vi "MiniReader.vi"() -> ()   [LabVIEW 2017]
uses:
  <vilib>/S3DK/PMU Recorder Light/PMU Recorder Light.lvlib
panel:
  out "error out":errorcluster
  in  "error in (no error)":errorcluster
  out "Buffer Active":bool
  out "Configuration File Received":bool
  out "Connected":bool
  out "Status Loop":bool
  out "Error":bool
  in  "Tab Control":T1(tab)
  out "Frequency":waveform(sgl)[](graph)
  out "Phasor_Mag":waveform(sgl)[](graph) caption="Frequency"
  out "Phasor_Ang":waveform(sgl)[](graph) caption="Frequency"
  out "Timestamp":timestamp[](array[timestamp])
  out "Analog Signals":sgl[][](array[numeric])
  out "Phasor Signals":csg[][](array[numeric])
  out "Digital Signals":bool[][](array[boolean])
  out "Has New Data?":bool
  out "Timed Loop":bool
  out "Signal Names":T2
  in  "Refresh Rate":i64(ring)=200 items=["50 Hz"=20, "20 Hz"=50, "10 Hz"=100, "5 Hz"=200, "2 Hz"=500, "1 Hz"=1000, "Every 2 sec"=2000, "Every 5 sec"=5000, "Every 10 sec"=10000, "Every minute"=60000]
  out "Quitting":bool
  in  "Activate PRL Read":bool=TRUE
  out "Execution Loop":bool
  out "Status":string
  in  "Channel Selector":bool
  in  "PRL Visible":bool
  in  "Quit":bool
  out "Event Loop":bool
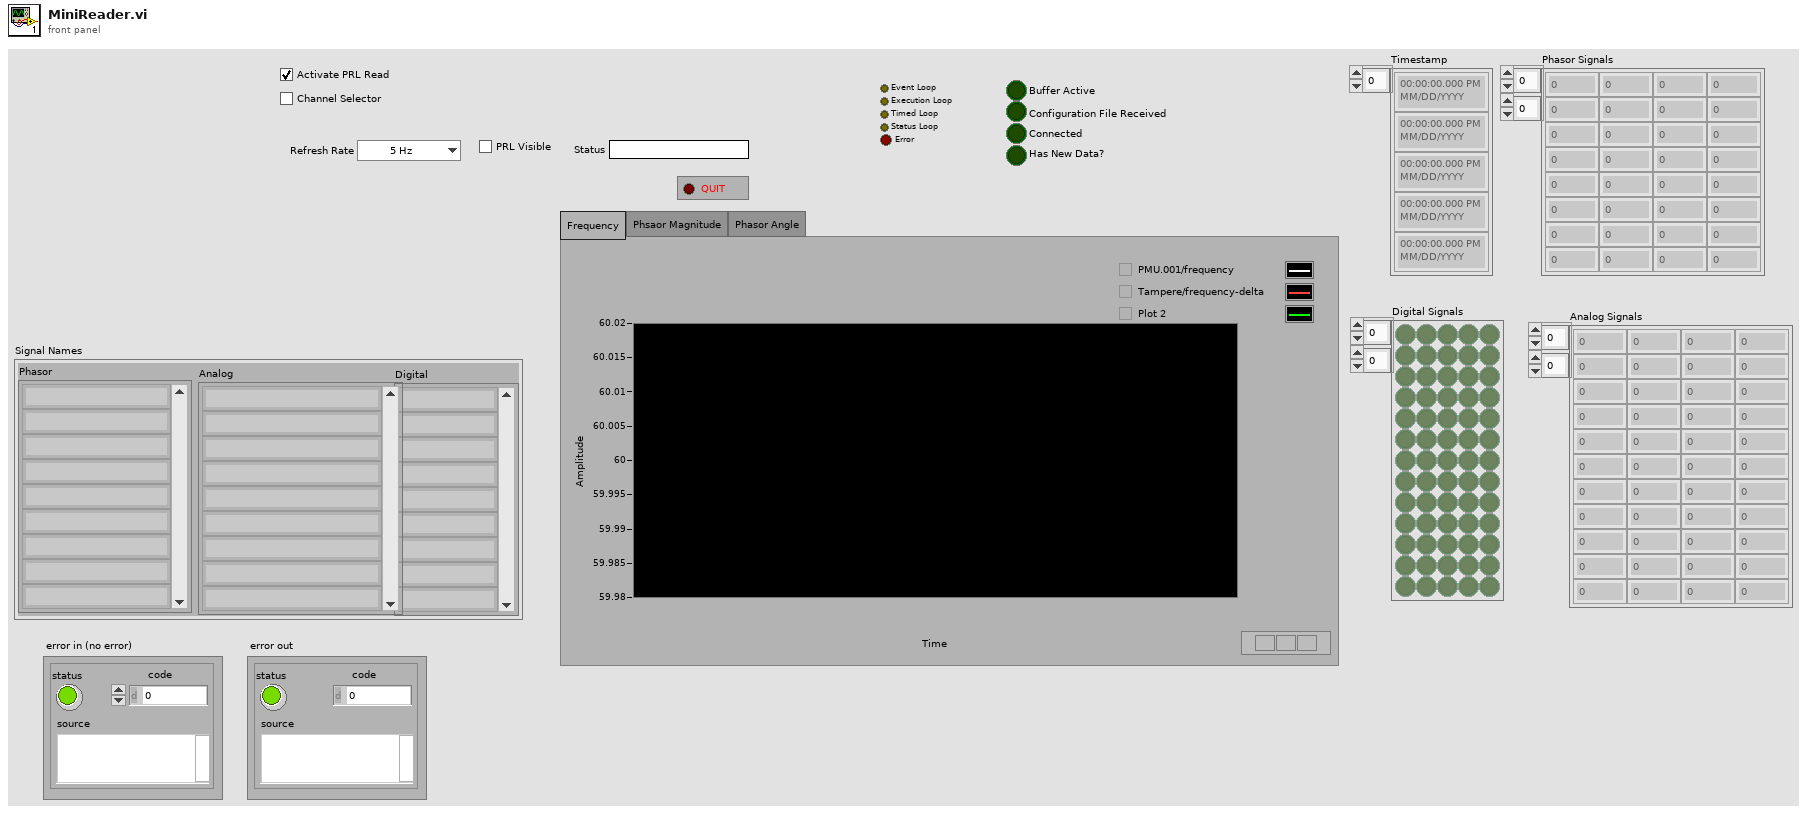
[diagram p1: front panel]
types:
  T1 = enum32{"Frequency", "Phsaor Magnitude", "Phasor Angle"}
  T2 = cluster{"Phasor":string[], "Analog":string[], "Digital":string[]}
  T3 = enum16{"Run", "Startup", "Get Status", "Pause", "Continue", "Shutdown", "Abort", "Open Panel", "Close Panel"}
  T4 = enum32{"Invalid", "Standard", "Closed", "Hidden", "Minimized", "Maximized"}
  T5 = enum16{"Filter Signals", "Get All Signal Names", "Select Signals on Name", "Select Frequency Only", "Get Selected Signal Names"}
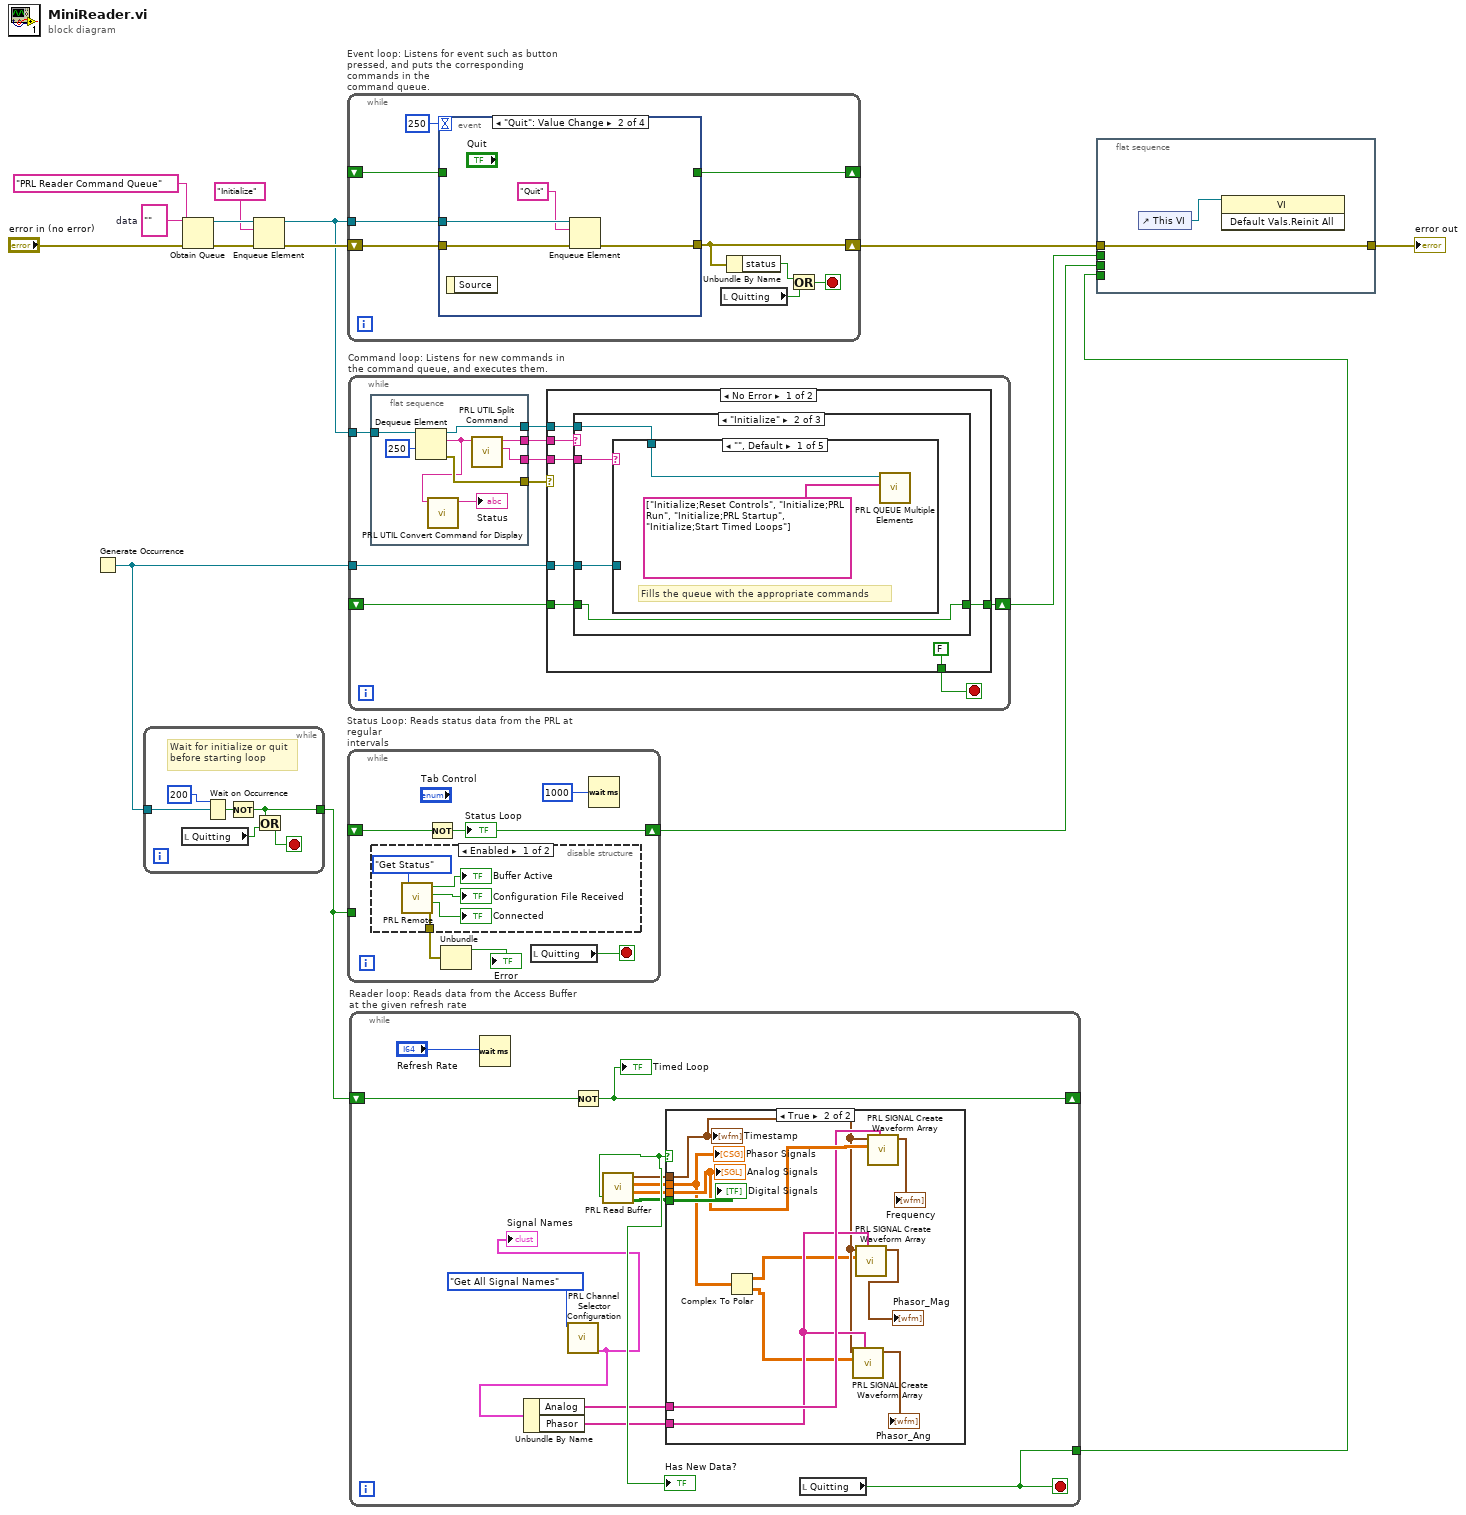
[diagram p0: block diagram]
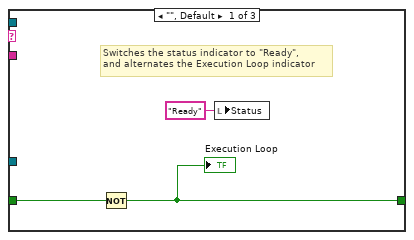
[diagram p4: hidden frame]
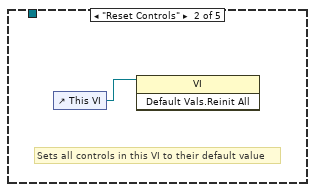
[diagram p5: hidden frame]
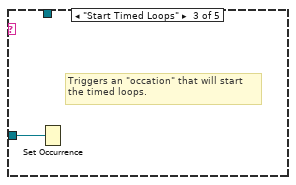
[diagram p6: hidden frame]
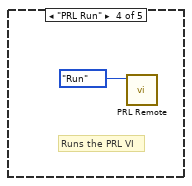
[diagram p7: hidden frame]
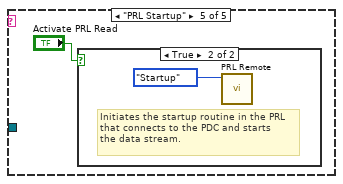
[diagram p8: hidden frame]
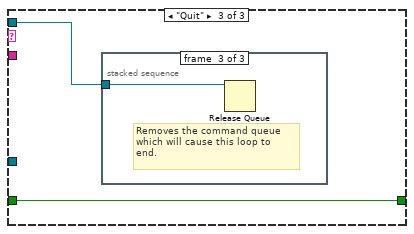
[diagram p10: hidden frame]
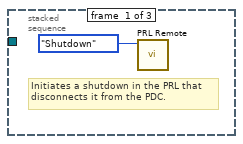
[diagram p11: hidden frame]
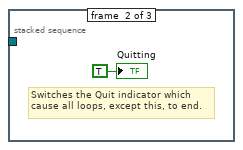
[diagram p12: hidden frame]
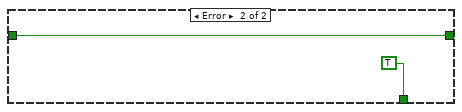
[diagram p13: hidden frame]
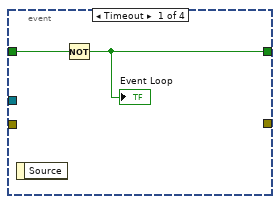
[diagram p14: hidden frame]
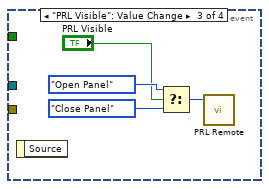
[diagram p15: hidden frame]
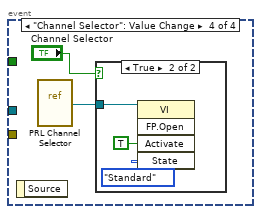
[diagram p16: hidden frame]
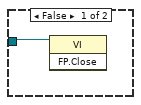
[diagram p17: hidden frame]
diagram:
  w15 = ""  # data
  n1 = Generate Occurrence() -> (w10:refnum<k4>)
  n2 = while {
    tunnel: w10 -> [w21]
    tunnel: [w16] -> w8
    stop <- w17 stop-if-true
    # "Wait for initialize or quit\nbefore starting loop"
    n3 = local read "Quitting"() -> (w18:bool)
    n4 = Wait on Occurrence(2:w21, 3:200 ("ms timeout (-1)")) -> (0:w19:bool)  [unwired: 1 in]
    n5 = Not(x=w19) -> (.not. x?=w16:bool)
    n6 = Or(x=w16, y=w18) -> (x .or. y?=w17:bool)
  }
  n7 = Obtain Queue(name (unnamed)="PRL Reader Command Queue", element data type=w15, error in (no error)="error in (no error)") -> (queue out=w14:refnum<queue>, error out=w13:errorcluster)  [unwired: 2 in, 1 out]
  n8 = Enqueue Element(queue=w14, element="Initialize", error in (no error)=w13) -> (queue out=w9:refnum<queue>, error out=w12:errorcluster)  [unwired: 1 in, 1 out]
  n9 = while "Event loop: Listens for event such as button pressed, and puts the corresponding commands in the\ncommand queue." {
    shift-right: [w27] -> w6
    shift-left: w12 -> [w29]
    tunnel: w9 -> [w30]
    shift-right: [w22] -> _
    shift-left: _ -> [w23]
    stop <- w28 stop-if-true
    n10 = event shown="[1] \"Quit\": Value Change" {
      selector: _ -> [_ _ _ _]
      dyn-events: _ -> [_ _ _ _]
      timeout: 250 -> [_ _ _ _]
      tunnel: w30 -> [_ w35 _ _]
      tunnel: w29 -> [_ w36 _ _]
      tunnel: [_ w34 _ _] -> w27
      tunnel: w23 -> [w32 _ _ _]
      tunnel: [w31 _ _ _] -> w22
      event Timeout {
        n11 = event-data() -> ()  [unwired: 1 in, 1 out]
        n12 = Not(x=w32) -> (.not. x?=w31:bool)
        "Event Loop" <- w31
      }
      event "Quit": Value Change {
        n13 = event-data() -> ()  [unwired: 1 in, 1 out]
        n14 = Enqueue Element(queue=w35, element="Quit", error in (no error)=w36) -> (error out=w34:errorcluster)  [unwired: 1 in, 2 out]
      }
      event "PRL Visible": Value Change {
        n15 = event-data() -> ()  [unwired: 1 in, 1 out]
        n16 = Select(t=T3."Open Panel" ("Action"), s="PRL Visible", f=T3."Close Panel" ("Action")) -> (s? t:f=w37:T3)
        n17 = call <vilib>:"PRL Remote.vi"("Action"=w37) -> ()  [unwired: 5 in, 6 out]
      }
      event "Channel Selector": Value Change {
        n18 = event-data() -> ()  [unwired: 1 in, 1 out]
        n19 = vi-ref <vilib>:"PRL Channel Selector.vi"() -> (w42:refnum<vi>)
        n20 = case shown="True" "Channel Selector" {
          tunnel: w42 -> [w43 w46]
          frame False {
            n21 = invoke class="VI" method="FP.Close"(reference=w43) -> ()  [unwired: 2 in, 3 out]
          }
          frame True {
            n22 = invoke class="VI" method="FP.Open"(reference=w46, "Activate"=TRUE ("Activate?"), "State"=T4."Standard") -> ()  [unwired: 2 in, 5 out]
          }
        }
      }
    }
    n23 = local read "Quitting"() -> (w24:bool)
    n24 = Unbundle By Name(w27) -> ("status"=w26:bool)
    n25 = Or(x=w26, y=w24) -> (x .or. y?=w28:bool)
  }
  n26 = while "Status Loop: Reads status data from the PRL at regular\nintervals" {
    tunnel: w8 -> [_]
    shift-right: [w50] -> w4
    shift-left: _ -> [w51]
    stop <- w52 stop-if-true
    n27 = disable-structure shown="Enabled" {
      disable-tunnel: [w53 _] -> w49
      frame Enabled {
        n28 = call <vilib>:"PRL Remote.vi"("Action"=T3."Get Status") -> ("error out"=w53:errorcluster, "Connected"=→"Connected":bool, "Configuration File Received"=→"Configuration File Received":bool, "Buffer Active"=→"Buffer Active":bool)  [unwired: 5 in, 2 out]
      }
      frame Disabled {
      }
    }
    n29 = Not(x=w51) -> (.not. x?=w50:bool)
    "Status Loop" <- w50
    n30 = Unbundle(w49) -> ("status"=→"Error":bool)  [unwired: 2 out]
    n31 = local read "Quitting"() -> (w52:bool)
    n32 = Wait (ms)(milliseconds to wait=i64 1000 ("Period")) -> ()  [unwired: 1 out]
  }
  n33 = while "Command loop: Listens for new commands in the command queue, and executes them." {
    tunnel: w9 -> [w66]
    tunnel: w10 -> [w63]
    shift-right: [w58] -> w5
    shift-left: _ -> [w59]
    stop <- w61 stop-if-true
    n34 = flat-sequence {
      tunnel: w66 -> [w74]
      tunnel: [w73] -> w65
      tunnel: [w72] -> w64
      tunnel: [w70] -> w62
      tunnel: [w67] -> w60
      frame #0 {
        n35 = Dequeue Element(queue=w74, timeout in ms (-1)=250) -> (queue out=w72:refnum<queue>, element=w69:string, error out=w73:errorcluster)  [unwired: 1 in, 1 out]
        n36 = call <vilib>:"PRL UTIL Convert Command for Display.vi"("Command In"=w69) -> ("Command Out"=→"Status":string)  [unwired: 10 in]
        n37 = call <vilib>:"PRL UTIL Split Command.vi"("Command"=w69) -> ("Parameters"=w67:string, "Command Out"=w70:string)  [unwired: 9 in]
      }
    }
    n38 = case shown="No Error" w65 {
      tunnel: w62 -> [w81 _]
      tunnel: w64 -> [w80 _]
      tunnel: w63 -> [w79 _]
      tunnel: [FALSE TRUE] -> w61
      tunnel: w60 -> [w77 _]
      tunnel: w59 -> [w76 w101]
      tunnel: [w75 w101] -> w58
      frame No Error {
        n39 = case shown="\"Initialize\"" w81 {
          tunnel: w80 -> [_ w87 w96]
          tunnel: w79 -> [_ w86 _]
          tunnel: w77 -> [_ w88 _]
          tunnel: w76 -> [w83 w85 w97]
          tunnel: [w82 w85 w97] -> w75
          frame "", Default {
            # "Switches the status indicator to \"Ready\",\nand alternates the Execution Loop indicator"
            n40 = Not(x=w83) -> (.not. x?=w82:bool)
            "Execution Loop" <- w82
            n41 = local write "Status"("Ready" ("Status")) -> ()
          }
          frame "Initialize" {
            n42 = case shown="\"\", Default" w88 {
              tunnel: w87 -> [w90 _ _ _ _]
              tunnel: w86 -> [_ _ w92 _ _]
              frame "", Default {
                # "Fills the queue with the appropriate commands"
                n43 = call <vilib>:"PRL QUEUE Multiple Elements.vi"("Elements to Add"=string[] ["Initialize;Reset Controls", "Initialize;PRL Run", "Initialize;PRL Startup", "Initialize;Start Timed Loops"], "queue"=w90) -> ()  [unwired: 8 in, 2 out]
              }
              frame "Reset Controls" {
                # "Sets all controls in this VI to their default value"
                n44 = control-ref of="This VI"() -> (w91:refnum<vi>)
                n45 = invoke class="VI" method="Default Vals.Reinit All"(reference=w91) -> ()  [unwired: 2 in, 3 out]
              }
              frame "Start Timed Loops" {
                # "Triggers an \"occation\" that will start \nthe timed loops."
                n46 = Set Occurrence(w92) -> ()
              }
              frame "PRL Run" {
                # "Runs the PRL VI"
                n47 = call <vilib>:"PRL Remote.vi"("Action"=T3."Run") -> ()  [unwired: 5 in, 6 out]
              }
              frame "PRL Startup" {
                n48 = case shown="True" "Activate PRL Read" {
                  frame False {
                  }
                  frame True {
                    # "Initiates the startup routine in the PRL\nthat connects to the PDC and starts\nthe data stream."
                    n49 = call <vilib>:"PRL Remote.vi"("Action"=T3."Startup") -> ()  [unwired: 5 in, 6 out]
                  }
                }
              }
            }
          }
          frame "Quit" {
            n50 = stacked-sequence {
              tunnel: w96 -> [_ _ w100]
              frame #0 {
                # "Initiates a shutdown in the PRL that\ndisconnects it from the PDC."
                n51 = call <vilib>:"PRL Remote.vi"("Action"=T3."Shutdown") -> ()  [unwired: 5 in, 6 out]
              }
              frame #1 {
                # "Switches the Quit indicator which\ncause all loops, except this, to end."
                "Quitting" <- TRUE ("Quitting")
              }
              frame #2 {
                # "Removes the command queue\nwhich will cause this loop to\nend."
                n52 = Release Queue(queue=w100) -> ()  [unwired: 2 in, 3 out]
              }
            }
          }
        }
      }
      frame Error {
      }
    }
  }
  n53 = while "Reader loop: Reads data from the Access Buffer at the given refresh rate" {
    tunnel: [w115] -> w1
    shift-right: [w104] -> _
    shift-left: w8 -> [w105]
    stop <- w115 stop-if-true
    n54 = Wait (ms)(milliseconds to wait="Refresh Rate") -> ()  [unwired: 1 out]
    n55 = call <vilib>:"PRL Channel Selector Configuration.vi"("Action"=T5."Get All Signal Names") -> ("Signal Names Out"=w106:T2)  [unwired: 10 in]
    "Signal Names" <- w106
    n56 = Unbundle By Name(w106) -> ("Analog"=w108:string[], "Phasor"=w107:string[])
    n57 = Not(x=w105) -> (.not. x?=w104:bool)
    "Timed Loop" <- w104
    n58 = call <vilib>:"PRL Read Buffer .vi"() -> ("Digital Signals"=w110:bool[][], "Analog Signals"=w111:sgl[][], "Phasor Signals"=w112:csg[][], "Timestamp"=w113:timestamp[], "Has Data"=w114:bool)  [unwired: 6 in, 1 out]
    "Has New Data?" <- w114
    n59 = case shown="True" w114 {
      tunnel: w113 -> [_ w121]
      tunnel: w111 -> [_ w125]
      tunnel: w112 -> [_ w120]
      tunnel: w110 -> [_ w126]
      tunnel: w108 -> [_ w124]
      tunnel: w107 -> [_ w122]
      frame False {
      }
      frame True {
        n60 = Complex To Polar(r * e^(i*theta)=w120) -> (r=w119:sgl[][], theta=w118:sgl[][])
        n61 = call <vilib>:"PRL SIGNAL Create Waveform Array.vi"("Signal Names"=w122, "Analog Signals"=w118, "Timestamp"=w121) -> ("Waveform Array"=→"Phasor_Ang":waveform(sgl)[])  [unwired: 8 in]
        n62 = call <vilib>:"PRL SIGNAL Create Waveform Array.vi"("Signal Names"=w122, "Analog Signals"=w119, "Timestamp"=w121) -> ("Waveform Array"=→"Phasor_Mag":waveform(sgl)[])  [unwired: 8 in]
        n63 = call <vilib>:"PRL SIGNAL Create Waveform Array.vi"("Signal Names"=w124, "Analog Signals"=w125, "Timestamp"=w121) -> ("Waveform Array"=→"Frequency":waveform(sgl)[])  [unwired: 8 in]
        "Timestamp" <- w121
        "Analog Signals" <- w125
        "Phasor Signals" <- w120
        "Digital Signals" <- w126
      }
    }
    n64 = local read "Quitting"() -> (w115:bool)
  }
  n65 = flat-sequence {
    tunnel: w6 -> [w127]
    tunnel: w5 -> [_]
    tunnel: w4 -> [_]
    tunnel: w1 -> [_]
    tunnel: [w127] -> w2
    frame #0 {
      n66 = control-ref of="This VI"() -> (w128:refnum<vi>)
      n67 = invoke class="VI" method="Default Vals.Reinit All"(reference=w128) -> ()  [unwired: 2 in, 3 out]
    }
  }
  "error out" <- w2
